vi "Execute.vi"(8 "error in (no error)":errorcluster, 11 "Node in":refnum<class "bt_Parallel_Threaded.lvclass">) -> (0 "error out":errorcluster, 1 "Status":T1, 3 "Node out":refnum<class "bt_Parallel_Threaded.lvclass">)   [LabVIEW 2021, in "BT.lvlib" / "bt_Parallel_Threaded.lvclass"]
uses:
  bt_Parallel_Threaded.lvclass
  C:/Users/Tim/Documents/GitHub/LV_Behaviour_Tree/Source/Support/Nodes/Composites/abs_Parallel/bt_Parallel.lvclass
  abs_Node/Status.ctl
  bt_Parallel_Threaded.lvclass/bt_Parallel_Threaded.ctl
  abs_Parallel/bt_Parallel.lvclass/bt_Parallel.ctl
  abs_Parallel/Properties/Read Status Calculation.vi
  abs_Parallel/bt_Parallel.lvclass
  System/bt_System.lvclass
  abs_Node/bt_Node.lvclass
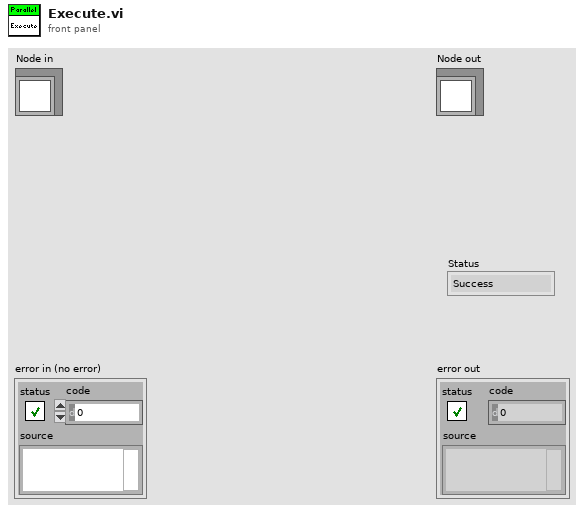
[diagram p1: front panel]
types:
  T1 = typedef "BT.lvlib/bt_Node.lvclass/Status.ctl" = enum16{"Success", "Failure", "Running"}
  T2 = typedef "Rendezvous RefNum" = refnum<k1>
  T3 = typedef "BT.lvlib/bt_Parallel.lvclass/Status Calculation.ctl" = enum16{"Succeed on All Succeed", "Failure on All Failure", "Succeed on Any Succeed", "Failure on Any Failure"}
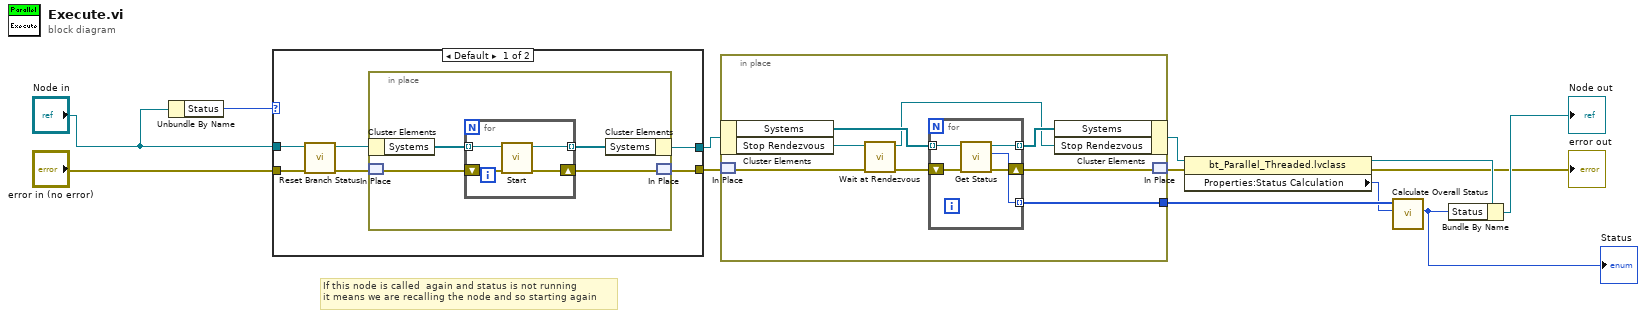
[diagram p0: block diagram]
diagram:
  # "If this node is called  again and status is not running\nit means we are recalling the node and so starting again"
  n1 = Unbundle By Name("Node in") -> ("Status"=w1:T1)
  n2 = case shown="Default" w1 {
    tunnel: [w15 w28] -> w9
    tunnel: [w14 w29] -> w8
    tunnel: "Node in" -> [w18 w29]
    tunnel: "error in (no error)" -> [w19 w28]
    frame Default {
      n3 = call "Reset Branch Status.vi"("error in (no error)"=w19, "bt_Parallel in"=w18) -> ("error out"=w16:errorcluster, "bt_Parallel out"=w17:refnum<class "bt_Parallel_Threaded.lvclass">)  [unwired: 8 in]
      n4 = in-place {
        n5 = in-place-cluster #1(w17) -> ("Systems"=w21:refnum<class "bt_System.lvclass">[])
        n6 = in-place-match #2(w16) -> (w20:errorcluster)
        n7 = for {
          tunnel: w21 -> [w27] mode=indexing
          tunnel: [w26] -> w23 mode=indexing
          shift-right: [w24] -> w22
          shift-left: w20 -> [w25]
          n8 = call "Start.vi"("error in (no error)"=w25, "bt_System in"=w27) -> ("error out"=w24:errorcluster, "bt_System out"=w26:refnum<class "bt_System.lvclass">)  [unwired: 8 in]
        }
        n9 = in-place-cluster #1("Systems"=w23) -> (w14:refnum<class "bt_Parallel_Threaded.lvclass">)
        n10 = in-place-match #2(w22) -> (w15:errorcluster)
      }
    }
    frame "Running" {
    }
  }
  n11 = in-place {
    in-place-border: [w36] -> w13
    n12 = in-place-cluster #3(w8) -> ("Systems"=w35:refnum<class "bt_System.lvclass">[], "Stop Rendezvous"=w31:T2)
    n13 = in-place-match #4(w9) -> (w33:errorcluster)
    n14 = call <vilib>:"Wait at Rendezvous.vi"("error in (no error)"=w33, "rendezvous"=w31) -> ("error out"=w32:errorcluster, "rendezvous out"=w30:T2)  [unwired: 3 in, 1 out]
    n15 = for {
      tunnel: [w40] -> w36 mode=indexing
      tunnel: w35 -> [w39] mode=indexing
      tunnel: [w38] -> w34 mode=indexing
      shift-right: [w41] -> w37
      shift-left: w32 -> [w42]
      n16 = call "Get Status.vi"("error in (no error)"=w42, "bt_System in"=w39) -> ("error out"=w41:errorcluster, "Status"=w40:T1, "bt_System out"=w38:refnum<class "bt_System.lvclass">)  [unwired: 7 in]
    }
    n17 = in-place-cluster #3("Systems"=w34, "Stop Rendezvous"=w30) -> (w11:refnum<class "bt_Parallel_Threaded.lvclass">)
    n18 = in-place-match #4(w37) -> (w12:errorcluster)
  }
  n19 = property class="bt_Parallel_Threaded.lvclass"(reference=w11, error in=w12) -> (reference out=w7:refnum<class "bt_Parallel_Threaded.lvclass">, error out=→"error out":errorcluster, "Properties:Status Calculation"=w10:T3)
  n20 = call "Calculate Overall Status.vi"("Status Calculation"=w10, "Status's"=w13) -> ("Overall Status"=w6:T1)  [unwired: 9 in]
  "Status" <- w6
  n21 = Bundle By Name(cluster=w7, "Status"=w6) -> (→"Node out":refnum<class "bt_Parallel_Threaded.lvclass">)
